vi "Inst_DAQ.vi"(8 "error in":errorcluster, 10 "All Message Queues in":T3, 11 "Prueba31 in":refnum<class "Prueba33.lvclass">) -> (0 "error out":errorcluster)   [LabVIEW 2019, in "Prueba33.lvclass"]
uses:
  Prueba33.lvclass
  QMH/Message Queue/All Message Queues.ctl
  QMH/Message Queue/Message Cluster.ctl
  Prueba33.lvclass/Prueba33.ctl
  <vilib>/DAQmx/read.llb/DAQmx Read (Analog 2D DBL NChan NSamp).vi
  <vilib>/Utility/error.llb/Error Cluster From Error Code.vi
  QMH/Message Queue/Enqueue Message (Single).vi
  <vilib>/DAQmx/miscellaneous.llb/DAQmx Fill In Error Info.vi
  <vilib>/ErrorRing/Error Ring.xnode
  QMH/Message Queue/Message Queue.lvlib
  Instrumento/CNT90/CNT90.lvclass
panel:
  out "AO Generador":T1(array[cluster])
  out "DetenerMonitor":T2
  out "SetDAQ_AO":T2
  out "GuardarVref":cluster{"Vref":dbl, "Channel":string}
  out "AjustarAmplitud":cluster{"Amplitud":dbl, "Channel":string}
  out "All States":string[](array[string])
  out "Actual State":string
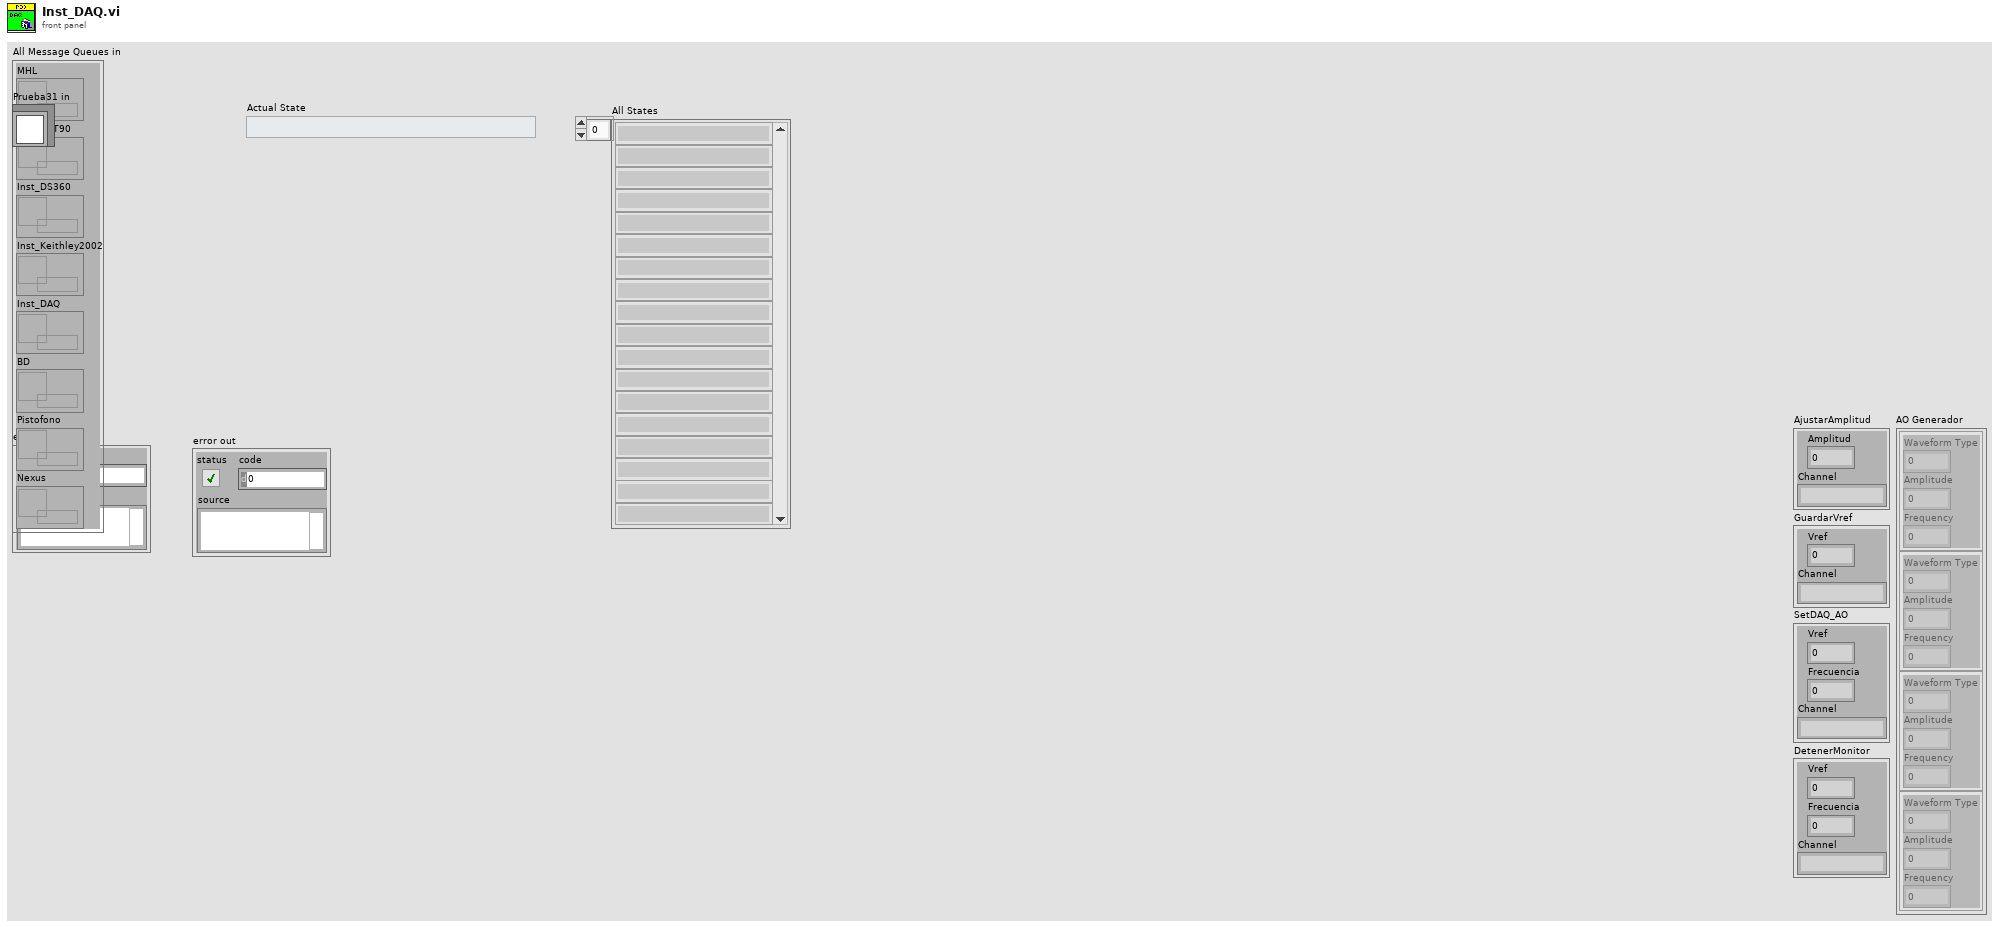
[diagram p1: front panel]
types:
  T1 = cluster{"Waveform Type":u16, "Amplitude":dbl, "Frequency":dbl}[]
  T2 = cluster{"Vref":dbl, "Frecuencia":dbl, "Channel":string}
  T3 = typedef "Message Queue.lvlib/All Message Queues.ctl" = cluster{"MHL":refnum<queue>, "Inst_CNT90":refnum<queue>, "Inst_DS360":refnum<queue>, "Inst_Keithley2002":refnum<queue>, "Inst_DAQ":refnum<queue>, "BD":refnum<queue>, "Pistofono":refnum<queue>, "Nexus":refnum<queue>}
  T4 = cluster{"Channel 1":cluster{"amplitude":dbl, "detected fundamental frequency":dbl}, "Channel 2":cluster{"amplitude":dbl, "detected fundamental frequency":dbl}, "Channel 3":cluster{"amplitude":dbl, "detected fundamental frequency":dbl}, "Channel 4":cluster{"amplitude":dbl, "detected fundamental frequency":dbl}}
  T5 = cluster{"Vref_D1":dbl, "Vref_D2":dbl, "Vref_D3":dbl, "Vref_D4":dbl}
  T6 = cluster{"amplitude":dbl, "detected fundamental frequency":dbl}
  T7 = cluster{"Waveform Type":u16, "Amplitude":dbl, "Frequency":dbl}
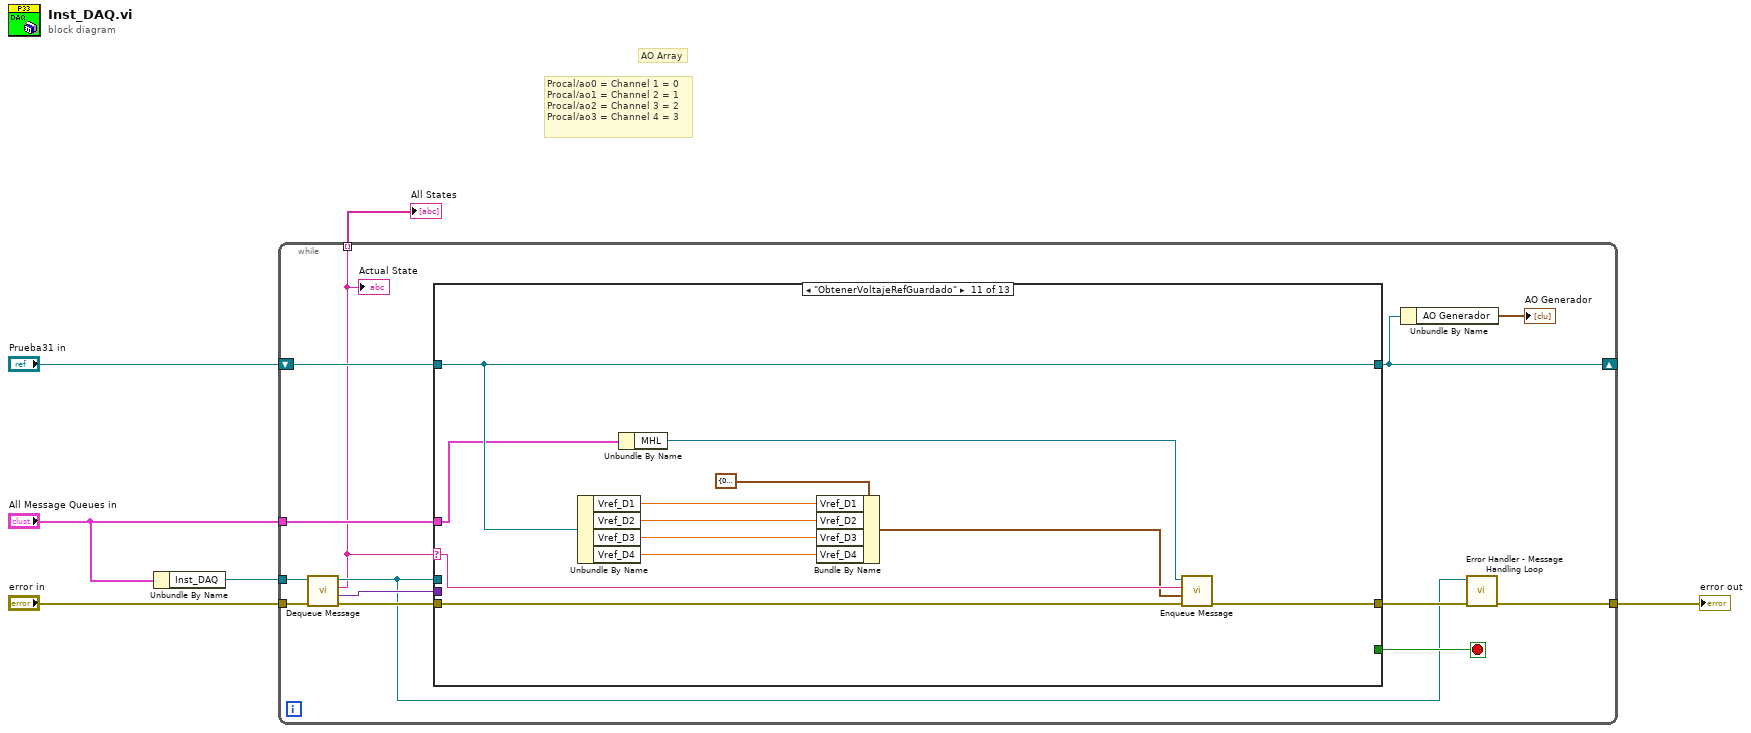
[diagram p0: block diagram]
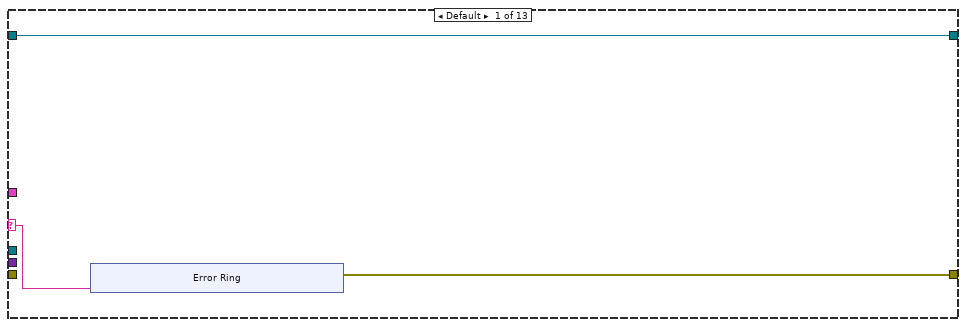
[diagram p2: hidden frame]
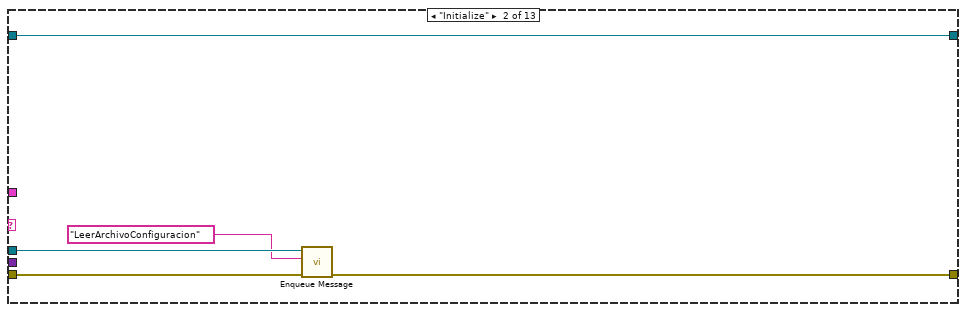
[diagram p3: hidden frame]
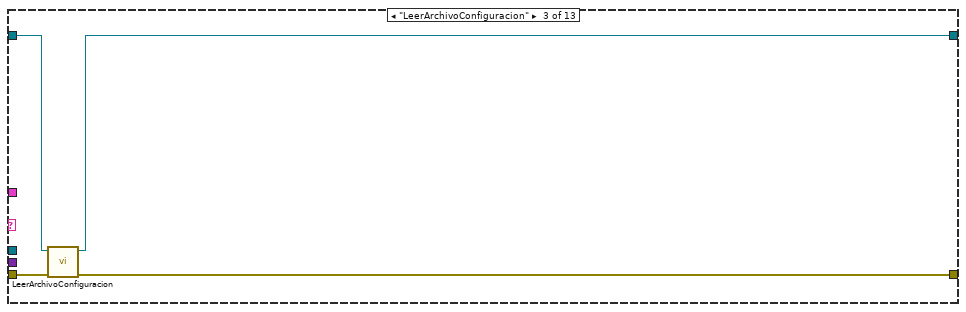
[diagram p4: hidden frame]
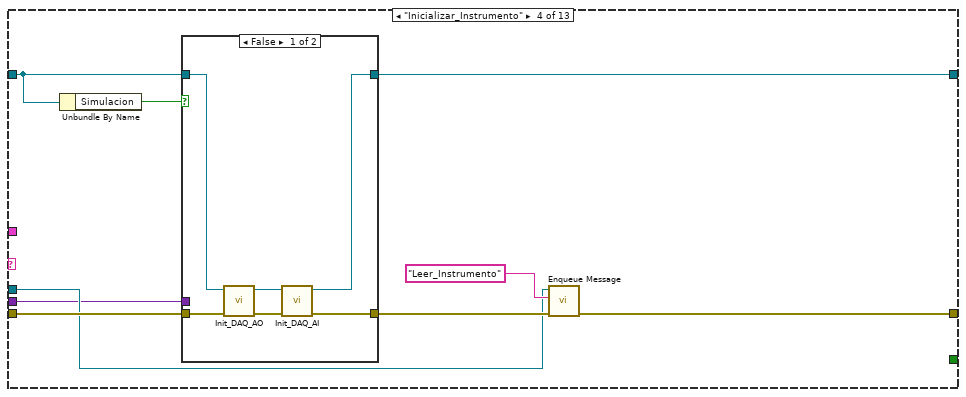
[diagram p5: hidden frame]
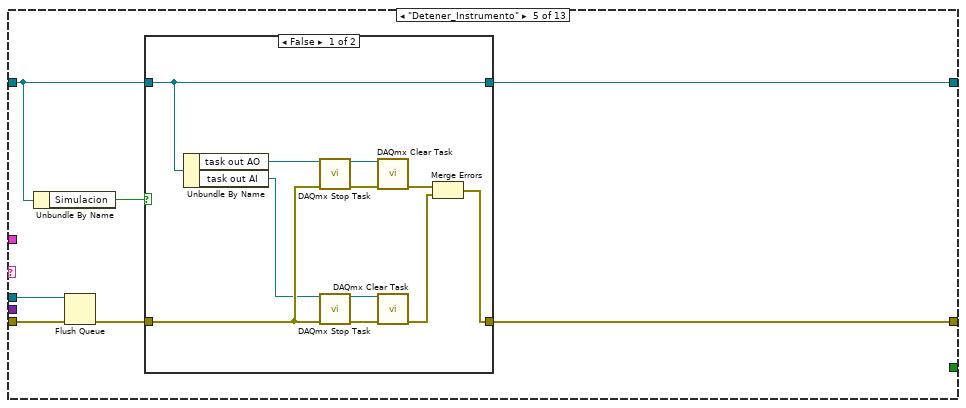
[diagram p7: hidden frame]
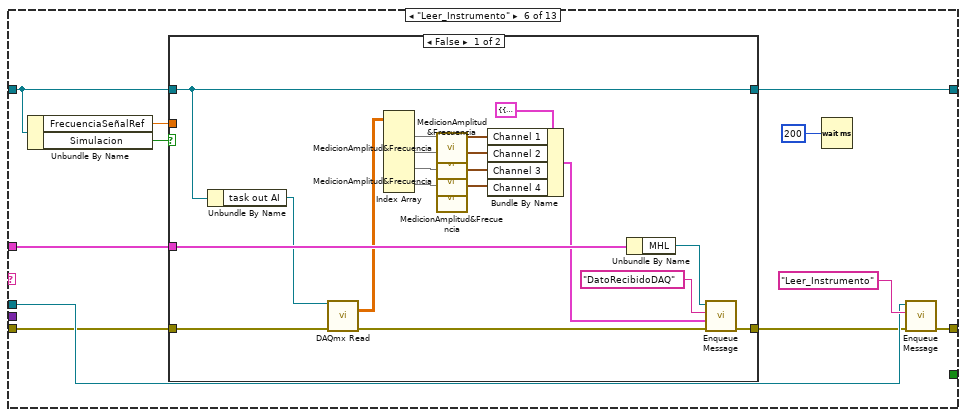
[diagram p9: hidden frame]
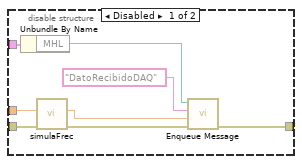
[diagram p11: hidden frame]
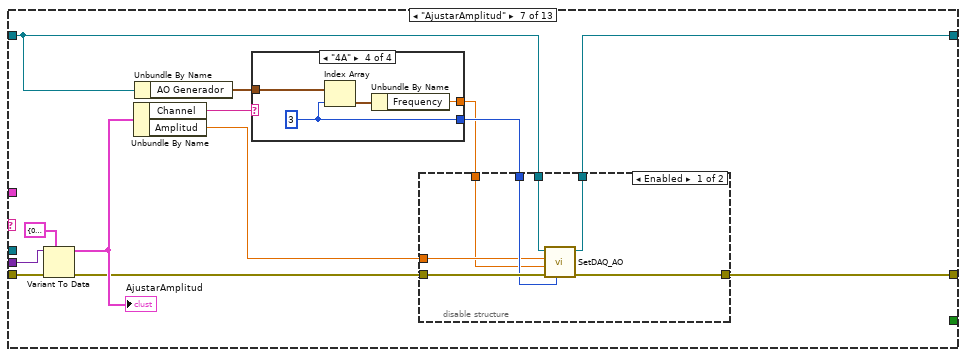
[diagram p12: hidden frame]
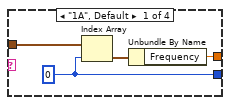
[diagram p14: hidden frame]
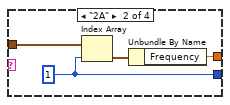
[diagram p15: hidden frame]
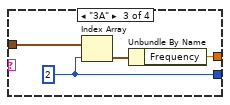
[diagram p16: hidden frame]
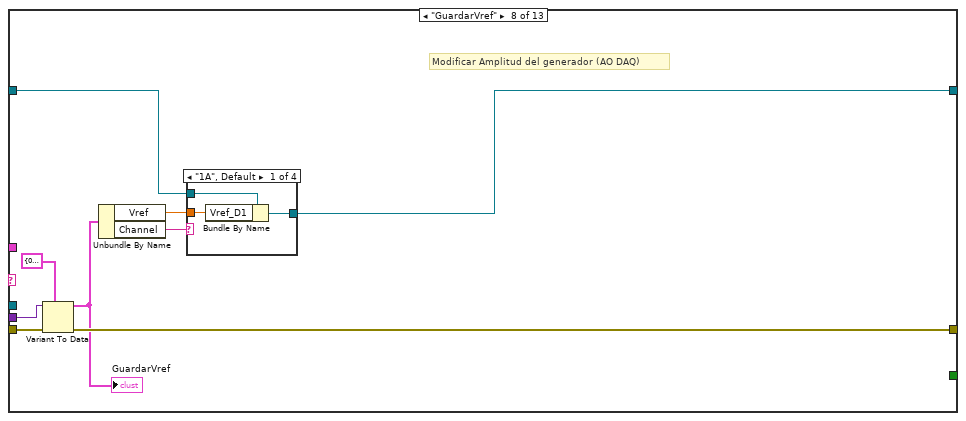
[diagram p17: hidden frame]
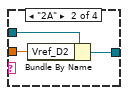
[diagram p18: hidden frame]
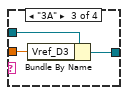
[diagram p19: hidden frame]
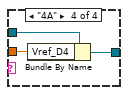
[diagram p20: hidden frame]
diagram:
  # "AO Array"
  # "Procal/ao0 = Channel 1 = 0\nProcal/ao1 = Channel 2 = 1\nProcal/ao2 = Channel 3 = 2\nProcal/ao3 = Channel 4 = 3"
  n1 = Unbundle By Name("All Message Queues in") -> ("Inst_DAQ"=w5:refnum<queue>)
  n2 = while {
    tunnel: "error in" -> [w19]
    tunnel: w5 -> [w18]
    tunnel: "All Message Queues in" -> [w17]
    tunnel: [w11] -> w3
    shift-right: [w8] -> _
    shift-left: "Prueba31 in" -> [w16]
    tunnel: [w9] -> w2 mode=indexing
    stop <- w13 stop-if-true
    n3 = call "Dequeue Message.vi"("error in (no error)"=w19, "Message Queue"=w18) -> ("error out"=w14:errorcluster, "Message Data"=w15:variant, "Message"=w9:string, "dup Message Queue"=w10:refnum<queue>)  [unwired: 6 in]
    "Actual State" <- w9
    n4 = case shown="\"ObtenerVoltajeRefGuardado\"" w9 {
      selector: w9 -> [w22 _ _ _ _ _ _ _ _ _ w237 w245 _]
      tunnel: w17 -> [_ _ _ _ _ w79 _ _ _ _ w230 w244 _]
      tunnel: w16 -> [w20 w30 w36 w40 w57 w76 w122 w159 w180 w218 w240 w242 w252]
      tunnel: w10 -> [_ w32 _ w42 w58 w84 _ _ _ _ _ _ w254]
      tunnel: w15 -> [_ _ _ w41 _ _ w131 w164 w191 w223 _ w248 _]
      tunnel: w14 -> [_ w33 w38 w47 w59 w82 w132 w165 w192 w224 w238 w249 w255]
      tunnel: [w21 w34 w35 w44 w62 w85 w126 w166 w182 w220 w239 w241 w251] -> w12
      tunnel: [w20 w30 w37 w39 w56 w77 w125 w160 w181 w219 w240 w242 w252] -> w8
      tunnel: [_ _ _ _ _ _ _ _ _ _ _ _ TRUE] -> w13
      frame Default {
        n5 = xnode "Error Ring"("parameter 0"=w22) -> ("error out"=w21:errorcluster)
      }
      frame "Initialize" {
        n6 = call-poly "Enqueue Message.vi"("error in (no error)"=w33, "Message"="LeerArchivoConfiguracion", "Message Queue"=w32) -> ("error out"=w34:errorcluster)  [unwired: 7 in, 1 out]
      }
      frame "LeerArchivoConfiguracion" {
        n7 = call "LeerArchivoConfiguracion.vi"("error in"=w38, "Prueba31 in"=w36) -> ("error out"=w35:errorcluster, "Prueba31 out"=w37:refnum<class "Prueba33.lvclass">)  [unwired: 8 in]
      }
      frame "Inicializar_Instrumento" {
        n8 = Unbundle By Name(w40) -> ("Simulacion"=w46:bool)
        n9 = case shown="False" w46 {
          tunnel: [w48 w55] -> w43
          tunnel: w47 -> [w52 w55]
          tunnel: w41 -> [_ _]
          tunnel: w40 -> [w53 w54]
          tunnel: [w49 w54] -> w39
          frame False {
            n10 = call "Init_DAQ_AO.vi"("error in"=w52, "Prueba31 in"=w53) -> ("error out"=w50:errorcluster, "Prueba31 out"=w51:refnum<class "Prueba33.lvclass">)  [unwired: 8 in]
            n11 = call "Init_DAQ_AI.vi"("error in (no error)"=w50, "Prueba33 in"=w51) -> ("error out"=w48:errorcluster, "Prueba33 out"=w49:refnum<class "Prueba33.lvclass">)  [unwired: 8 in]
          }
          frame True {
          }
        }
        n12 = call-poly "Enqueue Message.vi"("error in (no error)"=w43, "Message"="Leer_Instrumento", "Message Queue"=w42) -> ("error out"=w44:errorcluster)  [unwired: 7 in, 1 out]
      }
      frame "Detener_Instrumento" {
        n13 = Unbundle By Name(w57) -> ("Simulacion"=w61:bool)
        n14 = Flush Queue(queue=w58, error in (no error)=w59) -> (error out=w60:errorcluster)  [unwired: 2 out]
        n15 = case shown="False" w61 {
          tunnel: [w63 w75] -> w62
          tunnel: w60 -> [w69 w75]
          tunnel: [w66 w74] -> w56
          tunnel: w57 -> [w66 w74]
          frame False {
            n16 = Unbundle By Name(w66) -> ("task out AO"=w65:refnum<k21>, "task out AI"=w64:refnum<k21>)
            n17 = call <vilib>:"DAQmx Stop Task.vi"("task/channels in"=w65, "error in"=w69) -> ("task out"=w71:refnum<k21>, "error out"=w70:errorcluster)  [unwired: 12 in]
            n18 = call <vilib>:"DAQmx Stop Task.vi"("task/channels in"=w64, "error in"=w69) -> ("task out"=w72:refnum<k21>, "error out"=w73:errorcluster)  [unwired: 12 in]
            n19 = call <vilib>:"DAQmx Clear Task.vi"("task in"=w71, "error in"=w70) -> ("error out"=w68:errorcluster)  [unwired: 13 in]
            n20 = call <vilib>:"DAQmx Clear Task.vi"("task in"=w72, "error in"=w73) -> ("error out"=w67:errorcluster)  [unwired: 13 in]
            n21 = Merge Errors(w68, w67) -> (w63:errorcluster)
          }
          frame True {
          }
        }
      }
      frame "Leer_Instrumento" {
        n22 = Unbundle By Name(w76) -> ("FrecuenciaSeñalRef"=w78:dbl, "Simulacion"=w80:bool)
        n23 = case shown="False" w80 {
          tunnel: [w104 w110] -> w81
          tunnel: w82 -> [w100 w108]
          tunnel: w79 -> [w103 w109]
          tunnel: w78 -> [_ w107]
          tunnel: [w99 w106] -> w77
          tunnel: w76 -> [w99 w106]
          frame False {
            n24 = Unbundle By Name(w99) -> ("task out AI"=w98:refnum<k21>)
            n25 = call-poly <vilib>:"DAQmx Read.vi"("task/channels in"=w98, "error in"=w100) -> ("data"=w97:dbl[][], "error out"=w101:errorcluster)  [unwired: 11 in, 1 out]
            n26 = Index Array(array=w97) -> (element #1=w96:dbl[], element #2=w92:dbl[], element #3=w90:dbl[], element #4=w88:dbl[])  [unwired: 8 in]
            n27 = call "MedicionAmplitud&Frecuencia.vi"("data"=w96) -> ("Channel"=w94:T6)  [unwired: 10 in]
            n28 = call "MedicionAmplitud&Frecuencia.vi"("data"=w92) -> ("Channel"=w91:T6)  [unwired: 10 in]
            n29 = call "MedicionAmplitud&Frecuencia.vi"("data"=w90) -> ("Channel"=w89:T6)  [unwired: 10 in]
            n30 = call "MedicionAmplitud&Frecuencia.vi"("data"=w88) -> ("Channel"=w87:T6)  [unwired: 10 in]
            n31 = Bundle By Name(cluster=T4 {"Channel 1"={"amplitude"=0.0, "detected fundamental frequency"=0.0}, "Channel 2"={"amplitude"=0.0, "detected fundamental frequency"=0.0}, "Channel 3"={"amplitude"=0.0, "detected fundamental frequency"=0.0}, "Channel 4"={"amplitude"=0.0, "detected fundamental frequency"=0.0}}, "Channel 1"=w94, "Channel 2"=w91, "Channel 3"=w89, "Channel 4"=w87) -> (w93:T4)
            n32 = Unbundle By Name(w103) -> ("MHL"=w102:refnum<queue>)
            n33 = call-poly "Enqueue Message.vi"("error in (no error)"=w101, "Message Data"=w93, "Message"="DatoRecibidoDAQ", "Message Queue"=w102) -> ("error out"=w104:errorcluster)  [unwired: 6 in, 1 out]
          }
          frame True {
            n34 = disable-structure shown="Enabled" {
              disable-tunnel: [w117 w119] -> w110
              disable-tunnel: w109 -> [w116 _]
              disable-tunnel: w108 -> [w114 w119]
              disable-tunnel: w107 -> [w111 _]
              frame Disabled {
                n35 = Unbundle By Name(w116) -> ("MHL"=w115:refnum<queue>)
                n36 = call "simulaFrec.vi"("error in (no error)"=w114, "frec in"=w111) -> ("error out"=w113:errorcluster, "frec out"=w112:dbl)  [unwired: 7 in, 1 out]
                n37 = call-poly "Enqueue Message.vi"("error in (no error)"=w113, "Message Data"=w112, "Message"="DatoRecibidoDAQ", "Message Queue"=w115) -> ("error out"=w117:errorcluster)  [unwired: 6 in, 1 out]
              }
              frame Enabled {
              }
            }
          }
        }
        n38 = Wait (ms)(milliseconds to wait=u32 200) -> ()  [unwired: 1 out]
        n39 = call-poly "Enqueue Message.vi"("error in (no error)"=w81, "Message"="Leer_Instrumento", "Message Queue"=w84) -> ("error out"=w85:errorcluster)  [unwired: 7 in, 1 out]
      }
      frame "AjustarAmplitud" {
        n40 = Variant To Data(error in=w132, type=cluster{"Amplitud":dbl, "Channel":string} {"Amplitud"=0.0, "Channel"=""}, Variant=w131) -> (data=w129:cluster{"Amplitud":dbl, "Channel":string}, error out=w127:errorcluster)
        "AjustarAmplitud" <- w129
        n41 = Unbundle By Name(w129) -> ("Channel"=w128:string, "Amplitud"=w123:dbl)
        n42 = Unbundle By Name(w122) -> ("AO Generador"=w121:T1)
        n43 = case shown="\"4A\"" w128 {
          tunnel: [w144 w148 w152 w156] -> w124
          tunnel: w121 -> [w145 w149 w153 w157]
          tunnel: [w142 w146 w150 w154] -> w120
          frame "1A", Default {
            w144 = 0
            n44 = Index Array(array=w145, index=w144) -> (element=w143:T7)
            n45 = Unbundle By Name(w143) -> ("Frequency"=w142:dbl)
          }
          frame "2A" {
            w148 = 1
            n46 = Index Array(array=w149, index=w148) -> (element=w147:T7)
            n47 = Unbundle By Name(w147) -> ("Frequency"=w146:dbl)
          }
          frame "3A" {
            w152 = 2
            n48 = Index Array(array=w153, index=w152) -> (element=w151:T7)
            n49 = Unbundle By Name(w151) -> ("Frequency"=w150:dbl)
          }
          frame "4A" {
            w156 = 3
            n50 = Index Array(array=w157, index=w156) -> (element=w155:T7)
            n51 = Unbundle By Name(w155) -> ("Frequency"=w154:dbl)
          }
        }
        n52 = disable-structure shown="Enabled" {
          disable-tunnel: w127 -> [w139 w140]
          disable-tunnel: [w138 w140] -> w126
          disable-tunnel: [w137 w141] -> w125
          disable-tunnel: w124 -> [w136 _]
          disable-tunnel: w123 -> [w135 _]
          disable-tunnel: w122 -> [w134 w141]
          disable-tunnel: w120 -> [w133 _]
          frame Enabled {
            n53 = call "SetDAQ_AO.vi"("Index"=w136, "error in (no error)"=w139, "Frecuencia"=w133, "Vref"=w135, "Prueba33 in"=w134) -> ("error out"=w138:errorcluster, "Prueba33 out"=w137:refnum<class "Prueba33.lvclass">)  [unwired: 5 in]
          }
          frame Disabled {
          }
        }
      }
      frame "GuardarVref" {
        # "Modificar Amplitud del generador (AO DAQ)"
        n54 = Variant To Data(error in=w165, type=cluster{"Vref":dbl, "Channel":string} {"Vref"=0.0, "Channel"=""}, Variant=w164) -> (data=w162:cluster{"Vref":dbl, "Channel":string}, error out=w166:errorcluster)
        "GuardarVref" <- w162
        n55 = Unbundle By Name(w162) -> ("Vref"=w158:dbl, "Channel"=w161:string)
        n56 = case shown="\"1A\", Default" w161 {
          tunnel: w159 -> [w169 w172 w175 w178]
          tunnel: [w168 w171 w174 w177] -> w160
          tunnel: w158 -> [w167 w170 w173 w176]
          frame "1A", Default {
            n57 = Bundle By Name(cluster=w169, "Vref_D1"=w167) -> (w168:refnum<class "Prueba33.lvclass">)
          }
          frame "2A" {
            n58 = Bundle By Name(cluster=w172, "Vref_D2"=w170) -> (w171:refnum<class "Prueba33.lvclass">)
          }
          frame "3A" {
            n59 = Bundle By Name(cluster=w175, "Vref_D3"=w173) -> (w174:refnum<class "Prueba33.lvclass">)
          }
          frame "4A" {
            n60 = Bundle By Name(cluster=w178, "Vref_D4"=w176) -> (w177:refnum<class "Prueba33.lvclass">)
          }
        }
      }
      frame "SetDAQ_AO" {
        n61 = Variant To Data(error in=w192, type=T2 {"Vref"=0.0, "Frecuencia"=0.0, "Channel"=""}, Variant=w191) -> (data=w188:T2, error out=w183:errorcluster)
        n62 = Unbundle By Name(w188) -> ("Channel"=w189:string, "Frecuencia"=w190:dbl)
        n63 = case shown="\"1A\", \"1B\", Default" w189 {
          tunnel: w180 -> [w197 w202 w207 w212]
          tunnel: w190 -> [_ _ _ _]
          tunnel: w188 -> [w196 w201 w206 w211]
          tunnel: [w194 w199 w204 w209] -> w185
          tunnel: [0 1 2 3] -> w179
          frame "1A", "1B", Default {
            n64 = Unbundle By Name(w197) -> ("Vref_D1"=w195:dbl)
            n65 = Bundle By Name(cluster=w196, "Vref"=w195) -> (w194:T2)
          }
          frame "2A", "2B" {
            n66 = Unbundle By Name(w202) -> ("Vref_D2"=w200:dbl)
            n67 = Bundle By Name(cluster=w201, "Vref"=w200) -> (w199:T2)
          }
          frame "3A", "3B" {
            n68 = Unbundle By Name(w207) -> ("Vref_D3"=w205:dbl)
            n69 = Bundle By Name(cluster=w206, "Vref"=w205) -> (w204:T2)
          }
          frame "4A", "4B" {
            n70 = Unbundle By Name(w212) -> ("Vref_D4"=w210:dbl)
            n71 = Bundle By Name(cluster=w211, "Vref"=w210) -> (w209:T2)
          }
        }
        "SetDAQ_AO" <- w185
        n72 = Unbundle By Name(w185) -> ("Vref"=w186:dbl, "Frecuencia"=w184:dbl)
        n73 = call "SetDAQ_AO.vi"("Index"=w179, "error in (no error)"=w183, "Frecuencia"=w184, "Vref"=w186, "Prueba33 in"=w180) -> ("error out"=w182:errorcluster, "Prueba33 out"=w181:refnum<class "Prueba33.lvclass">)  [unwired: 5 in]
      }
      frame "DetenerMonitor" {
        n74 = Variant To Data(error in=w224, type=T2 {"Vref"=0.0, "Frecuencia"=0.0, "Channel"=""}, Variant=w223) -> (data=w217:T2, error out=w221:errorcluster)
        "DetenerMonitor" <- w217
        n75 = Unbundle By Name(w217) -> ("Vref"=w216:dbl, "Frecuencia"=w215:dbl, "Channel"=w214:string)
        n76 = case shown="\"4A\", \"4B\"" w214 {
          tunnel: [0 1 2 3] -> w213
          frame "1A", "1B", Default {
          }
          frame "2A", "2B" {
          }
          frame "3A", "3B" {
          }
          frame "4A", "4B" {
          }
        }
        n77 = call "SetDAQ_AO.vi"("Index"=w213, "error in (no error)"=w221, "Frecuencia"=w215, "Vref"=w216, "Prueba33 in"=w218) -> ("error out"=w220:errorcluster, "Prueba33 out"=w219:refnum<class "Prueba33.lvclass">)  [unwired: 5 in]
      }
      frame "ObtenerVoltajeRefGuardado" {
        n78 = Unbundle By Name(w240) -> ("Vref_D1"=w235:dbl, "Vref_D2"=w234:dbl, "Vref_D3"=w233:dbl, "Vref_D4"=w232:dbl)
        n79 = Unbundle By Name(w230) -> ("MHL"=w229:refnum<queue>)
        n80 = Bundle By Name(cluster=T5 {"Vref_D1"=0.0, "Vref_D2"=0.0, "Vref_D3"=0.0, "Vref_D4"=0.0}, "Vref_D1"=w235, "Vref_D2"=w234, "Vref_D3"=w233, "Vref_D4"=w232) -> (w231:T5)
        n81 = call-poly "Enqueue Message.vi"("error in (no error)"=w238, "Message Data"=w231, "Message"=w237, "Message Queue"=w229) -> ("error out"=w239:errorcluster)  [unwired: 6 in, 1 out]
      }
      frame "Error" {
        n82 = Unbundle By Name(w244) -> ("MHL"=w243:refnum<queue>)
        n83 = Variant To Data(error in=w249, type=errorcluster {"status"=FALSE, "code"=0, "source"=""} ("error constant"), Variant=w248) -> (data=w246:errorcluster, error out=w247:errorcluster)
        n84 = call-poly "Enqueue Message.vi"("error in (no error)"=w247, "Message Data"=w246, "Message"=w245, "Message Queue"=w243) -> ("error out"=w241:errorcluster)  [unwired: 6 in, 1 out]
      }
      frame "Exit" {
        n85 = Release Queue(queue=w254, error in (no error)=w255) -> (error out=w251:errorcluster)  [unwired: 1 in, 2 out]
      }
    }
    n86 = Unbundle By Name(w8) -> ("AO Generador"=→"AO Generador":T1)
    n87 = call "Error Handler - Message Handling Loop.vi"("error in (no error)"=w12, "Message Queue"=w10) -> ("dup error in"=w11:errorcluster)  [unwired: 8 in, 1 out]
  }
  "error out" <- w3
  "All States" <- w2
